vi "Agilent SNA Set Message Mode.vi"(7 "Agilent SNA & SWP":T2, 8 "error in (no error)":errorcluster, 10 "Message Mode":T1, 11 "VISA Resource Names":T3) -> (0 "error out":errorcluster, 3 "dup VISA Resource Names":T3)   [LabVIEW 2011]
doc: "This VI for the HP8753B Network Analyzers reads the stimulus values. Except when performing log sweeps and freq list sweeps, this VI uses the start and stop values and the number of points to calcuate the stimulus values."
uses:
  TypeDefs/Agilent SNA VISA.ctl
  TypeDefs/Agilent SNA Instrument Info.ctl
  TypeDefs/Agilent SNA Message Mode.ctl
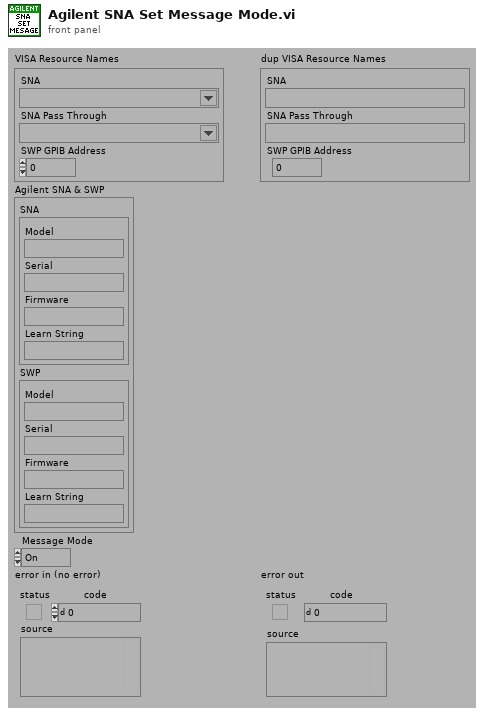
[diagram p1: front panel]
types:
  T1 = typedef "Agilent SNA Message Mode.ctl" = enum16{"On", "Off"}
  T2 = typedef "Agilent SNA Instrument Info.ctl" = cluster{"SNA":cluster{"Model":string, "Serial":string, "Firmware":string, "Learn String":string}, "SWP":cluster{"Model":string, "Serial":string, "Firmware":string, "Learn String":string}}
  T3 = typedef "Agilent SNA VISA.ctl" = cluster{"SNA":refnum<visa-resource-name>, "SNA Pass Through":refnum<visa-resource-name>, "SWP GPIB Address":i32}
  T4 = typedef "Agilent SNA Model.ctl" = enum16{"Not Supported", "8757X"}
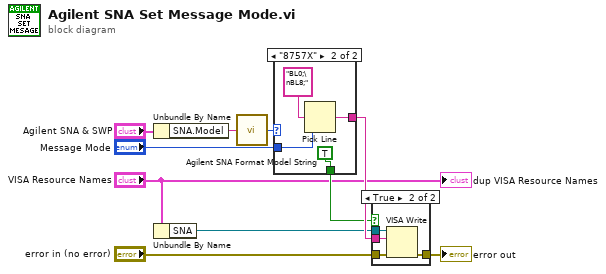
[diagram p0: block diagram]
diagram:
  n1 = Unbundle By Name("Agilent SNA & SWP") -> ("SNA.Model"=w4:string)
  n2 = Unbundle By Name("VISA Resource Names") -> ("SNA"=w2:refnum<visa-resource-name>)
  n3 = call "Agilent SNA Format Model String.vi"("Model String"=w4) -> ("Model"=w10:T4)
  n4 = case shown="\"8757X\"" w10 {
    tunnel: [_ w13] -> w8
    tunnel: "Message Mode" -> [_ w12]
    tunnel: [_ TRUE] -> w6
    frame "Not Supported" {
    }
    frame "8757X" {
      n5 = Pick Line(multi-line string="BL0;\nBL8;", line index=w12) -> (output string=w13:string)  [unwired: 1 out]
    }
  }
  n6 = case shown="True" w6 {
    tunnel: [w15 w19] -> w9
    tunnel: w8 -> [_ w18]
    tunnel: w2 -> [_ w17]
    tunnel: "error in (no error)" -> [w15 w16]
    frame False {
    }
    frame True {
      n7 = VISA Write(VISA resource name=w17, write buffer=w18, error in (no error)=w16) -> (error out=w19:errorcluster)  [unwired: 2 out]
    }
  }
  "error out" <- w9
  "dup VISA Resource Names" <- "VISA Resource Names"
